vi "LL_GET Bucket.vi"(7 "GET Bucket Request Parameters":T8 {"max-keys" max=1000}, 8 "error in (no error)":errorcluster, 9 "Bucket":string, 11 "Headers":T7[](array[typedef])) -> (0 "error out":errorcluster, 1 "Call Result":T1, 3 "ListBucketResult":T2)   [LabVIEW 2011, in "LV Interface for Amazon S3.lvlib"]
doc: "This core implementation of the GET operation returns some or all (up to 1000) of the objects in a bucket. You can use the request parameters as selection criteria to return a subset of the objects in a bucket. You have direct access to HTTP headers, so you can use this VI to implement special requests or API calls not present in this toolkit."
uses:
  LV Interface for Amazon S3.lvlib
  Typedefs/AMZ_S3_API_GET Bucket Request Parameters.ctl
  Typedefs/AMZ_S3_HTTP Header-Value pair.ctl
  Typedefs/AMZ_S3_API_ListBucketResult.ctl
  Typedefs/AMZ_S3_API_ListBucketResult Content.ctl
  Typedefs/AMZ_S3_Storage Class.ctl
  Typedefs/AMZ_S3_API_Owner.ctl
  Typedefs/AMZ_S3_API_ListBucketResult CommonPrefix.ctl
  Typedefs/AMZ_S3_Call Results.ctl
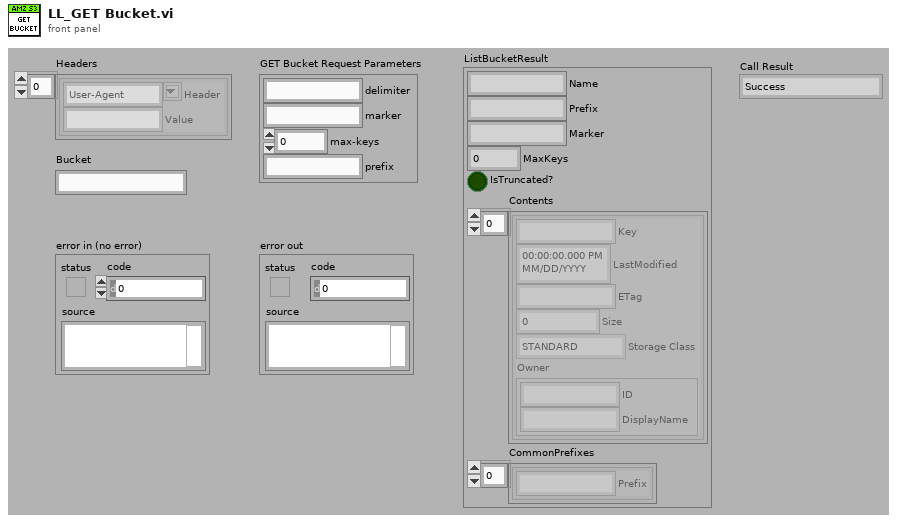
[diagram p1: front panel]
types:
  T1 = typedef "LV Interface for Amazon S3.lvlib/AMZ_S3_Call Results.ctl" = enum16{"Success", "UndefinedError", "AccessDenied", "AccountProblem", "AmbiguousGrantByEmailAddress", "BadDigest", "BucketAlreadyExists", "BucketAlreadyOwnedByYou", "BucketNotEmpty", "CredentialsNotSupported", "CrossLocationLoggingProhibited", "EntityTooSmall", "EntityTooLarge", "ExpiredToken", "IllegalVersioningConfigurationException", "IncompleteBody", "IncorrectNumberOfFilesInPostRequest", "InlineDataTooLarge", "InternalError", "InvalidAccessKeyId", "InvalidAddressingHeader", "InvalidArgument", "InvalidBucketName", "InvalidDigest", "InvalidLocationConstraint", "InvalidPart", "InvalidPartOrder", "InvalidPayer", "InvalidPolicyDocument", "InvalidRange", "InvalidSecurity", "InvalidSOAPRequest", "InvalidStorageClass", "InvalidTargetBucketForLogging", "InvalidToken", "InvalidURI", "KeyTooLong", "MalformedACLError", "MalformedPOSTRequest", "MalformedXML", "MaxMessageLengthExceeded", "MaxPostPreDataLengthExceededError", "MetadataTooLarge", "MethodNotAllowed", "MissingAttachment", "MissingContentLength", "MissingRequestBodyError", "MissingSecurityElement", "MissingSecurityHeader", "NoLoggingStatusForKey", "NoSuchBucket", "NoSuchKey", "NoSuchUpload", "NoSuchVersion", "NotImplemented", "NotSignedUp", "OperationAborted", "PermanentRedirect", "PreconditionFailed", "Redirect", "RequestIsNotMultiPartContent", "RequestTimeout", "RequestTimeTooSkewed", "RequestTorrentOfBucketError", "SignatureDoesNotMatch", "SlowDown", "TemporaryRedirect", "TokenRefreshRequired", "TooManyBuckets", "UnexpectedContent", "UnresolvableGrantByEmailAddress", "UserKeyMustBeSpecified", "LabVIEWError"}
  T2 = typedef "LV Interface for Amazon S3.lvlib/AMZ_S3_API_ListBucketResult.ctl" = cluster{"Name":string, "Prefix":string, "Marker":string, "MaxKeys":u16, "IsTruncated?":bool, "Contents":T3[], "CommonPrefixes":T6[]}
  T3 = typedef "LV Interface for Amazon S3.lvlib/AMZ_S3_API_ListBucketResult Content.ctl" = cluster{"Key":string, "LastModified":timestamp, "ETag":string, "Size":u64, "Storage Class":T4, "Owner":T5}
  T4 = typedef "LV Interface for Amazon S3.lvlib/AMZ_S3_Storage Class.ctl" = enum16{"STANDARD", "REDUCED_REDUNDANCY"}
  T5 = typedef "LV Interface for Amazon S3.lvlib/AMZ_S3_API_Owner.ctl" = cluster{"ID":string, "DisplayName":string}
  T6 = typedef "LV Interface for Amazon S3.lvlib/AMZ_S3_API_ListBucketResult CommonPrefix.ctl" = cluster{"Prefix":string}
  T7 = typedef "LV Interface for Amazon S3.lvlib/AMZ_S3_HTTP Header-Value pair.ctl" = cluster{"Header":string, "Value":string}
  T8 = typedef "LV Interface for Amazon S3.lvlib/AMZ_S3_API_GET Bucket Request Parameters.ctl" = cluster{"delimiter":string, "marker":string, "max-keys":u16, "prefix":string}
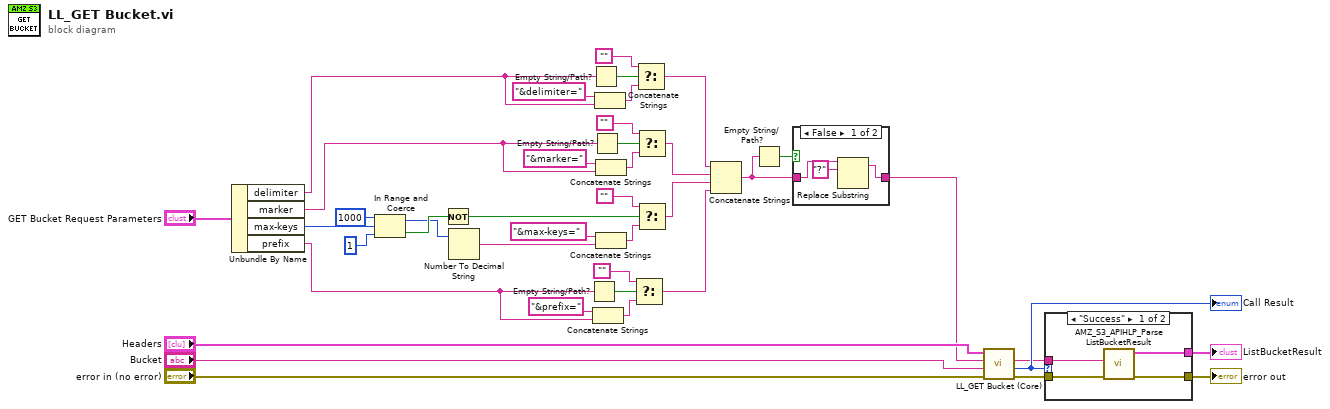
[diagram p0: block diagram]
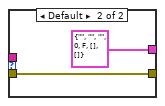
[diagram p2: hidden frame]
diagram:
  n1 = Unbundle By Name("GET Bucket Request Parameters") -> ("delimiter"=w17:string, "marker"=w16:string, "max-keys"=w7:u16, "prefix"=w15:string)
  n2 = In Range and Coerce(upper limit=u16 1000, x=w7, lower limit=u16 1) -> (coerced(x)=w2:u16, In Range?=w4:bool)
  n3 = Not(x=w4) -> (.not. x?=w3:bool)
  n4 = Number To Decimal String(number=w2) -> (decimal integer string=w29:string)  [unwired: 1 in]
  n5 = Empty String/Path?(string/path=w15) -> (empty?=w27:bool)
  n6 = Empty String/Path?(string/path=w17) -> (empty?=w38:bool)
  n7 = Empty String/Path?(string/path=w16) -> (empty?=w35:bool)
  n8 = Concatenate Strings("&prefix=" ("string"), w15) -> (w28:string)
  n9 = Concatenate Strings("&delimiter=" ("string"), w17) -> (w37:string)
  n10 = Concatenate Strings("&marker=" ("string"), w16) -> (w36:string)
  n11 = Concatenate Strings("&max-keys=" ("string"), w29) -> (w30:string)
  n12 = Select(t="", s=w27, f=w28) -> (s? t:f=w22:string)
  n13 = Select(t="", s=w38, f=w37) -> (s? t:f=w24:string)
  n14 = Select(t="", s=w35, f=w36) -> (s? t:f=w23:string)
  n15 = Select(t="", s=w3, f=w30) -> (s? t:f=w21:string)
  n16 = Concatenate Strings(w24, w23, w21, w22) -> (w20:string)
  n17 = Empty String/Path?(string/path=w20) -> (empty?=w19:bool)
  n18 = case shown="False" w19 {
    tunnel: w20 -> [w44 w45]
    tunnel: [w42 w45] -> w1
    frame False {
      n19 = Replace Substring(4:"?" ("substring (\"\")"), 5:w44) -> (1:w42:string)  [unwired: 2 in, 1 out]
    }
    frame True {
    }
  }
  n20 = call "LL_GET Bucket (Core).vi"("error in (no error)"="error in (no error)", "Bucket"="Bucket", "Path and query string"=w1, "Headers"="Headers") -> ("error out"=w10:errorcluster, "Call Result"=w12:T1, "Response body"=w11:string)  [unwired: 4 in, 1 out]
  "Call Result" <- w12
  n21 = case shown="\"Success\"" w12 {
    tunnel: w11 -> [w49 _]
    tunnel: w10 -> [w48 w50]
    tunnel: [w47 T2 {"Name"="", "Prefix"="", "Marker"="", "MaxKeys"=0, "IsTruncated?"=FALSE, "Contents"=[], "CommonPrefixes"=[]} ("ListBucketResult")] -> w9
    tunnel: [w46 w50] -> w8
    frame "Success" {
      n22 = call "AMZ_S3_APIHLP_Parse ListBucketResult.vi"("error in (no error)"=w48, "Response body"=w49) -> ("error out"=w46:errorcluster, "ListBucketResult"=w47:T2)  [unwired: 8 in]
    }
    frame Default {
    }
  }
  "ListBucketResult" <- w9
  "error out" <- w8
